vi "create_http_communication.vi"(0 "api_key":string, 11 "error in":errorcluster) -> (4 "client handle":T1, 15 "error out":errorcluster)   [LabVIEW 2020, in "vector_weviate.lvclass"]
doc: "This VI creates the HTTP request URL for Weviate Vector Store"
uses:
  vector_weviate.lvclass
  <vilib>/httpClient/ClientHandle.ctl
  <vilib>/httpClient/LabVIEWHTTPClient.lvlib
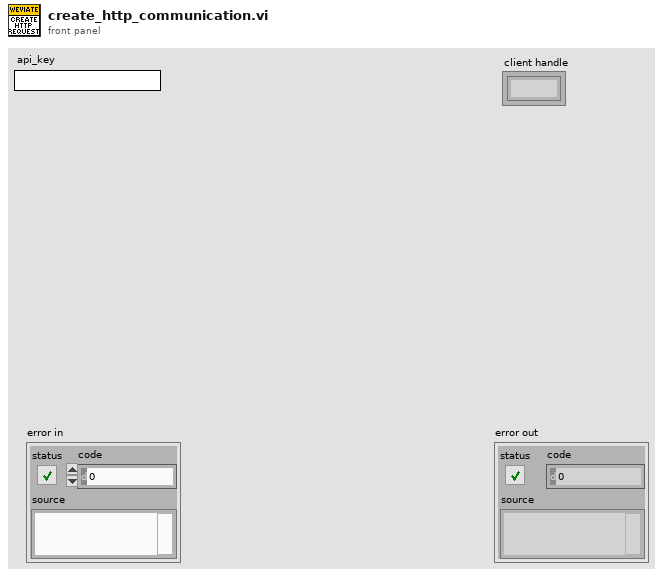
[diagram p1: front panel]
types:
  T1 = typedef "LabVIEWHTTPClient.lvlib/ClientHandle.ctl" = refnum<k1>
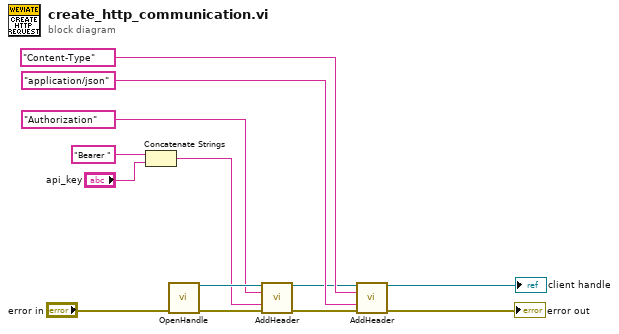
[diagram p0: block diagram]
diagram:
  n1 = Concatenate Strings("Bearer " ("string"), "api_key") -> (w1:string)
  n2 = call <vilib>:"OpenHandle.vi"("error in (no error)"="error in") -> ("client handle out"=w11:T1, "error out"=w12:errorcluster)  [unwired: 13 in]
  n3 = call <vilib>:"AddHeader.vi"("client handle"=w11, "header"="Authorization", "value"=w1, "error in (no error)"=w12) -> ("client handle out"=w5:T1, "error out"=w9:errorcluster)  [unwired: 10 in]
  n4 = call <vilib>:"AddHeader.vi"("client handle"=w5, "header"="Content-Type", "value"="application/json", "error in (no error)"=w9) -> ("client handle out"=→"client handle":T1, "error out"=→"error out":errorcluster)  [unwired: 10 in]
